vi "CustomDataHelperIAFLCytometer.vi"(0 "object in":refnum<class "AD2_DO_SDK.lvclass">, 2 "Pulse Settings":T1, 5 "error in (no error)":errorcluster) -> (14 "object out":refnum<class "AD2_DO_SDK.lvclass">, 19 "error out":errorcluster)   [LabVIEW 2019, in "AD2_DO_SDK.lvclass"]
doc: "This VI doest the same as DOconfigureCustomPattern but With a different Front panel. It is custom-made for the IAF Cytometer application"
uses:
  AD2_DO_SDK.lvclass
  DOConfigureCustomData.ctl
  DOTrigger.ctl
  AD2_WFG_SDK_class/AD2TriggerSources.ctl
  DOCustomData.ctl
  AD2_SDK_class/AD2_SDK.lvclass
panel:
  out "Numeric":i32
  out "Array 2":bool[](array[boolean])
  out "Array":bool[][](array[boolean])
  out "x*y":dbl[](array[numeric])
  # "DIO0 (camera)"
  # "DIO1 (COOL-LED CH1)"
  # "DIO2 (COOL-LED CH2)"
  # "DIO3 (COOL-LED CH1)"
  # "DIO0 Pulses at the same time as DIO1,2 and 3 +-offset"
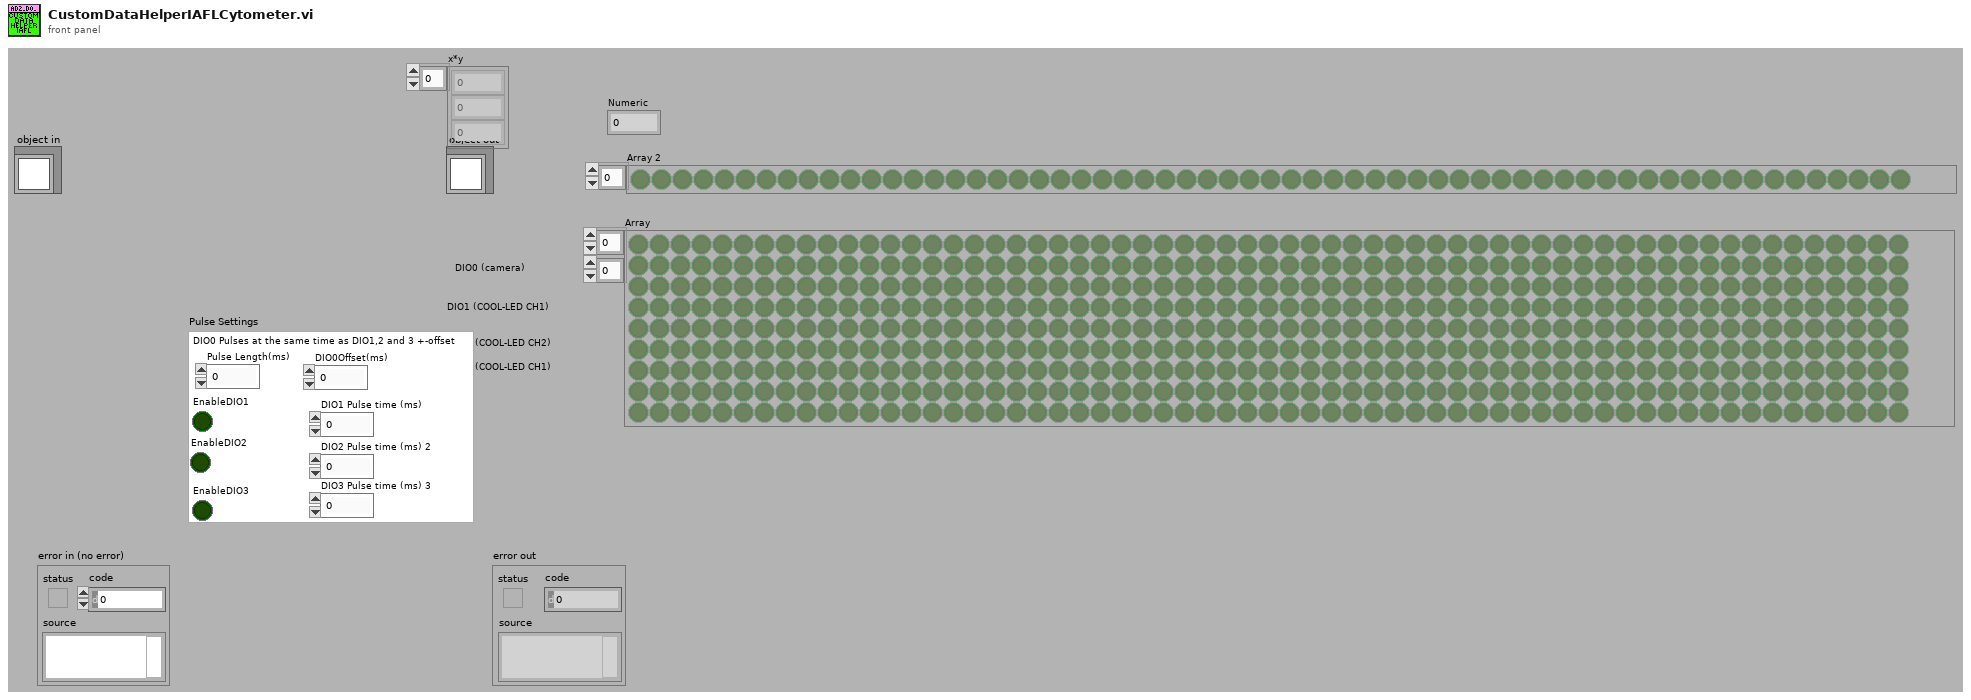
[diagram p1: front panel]
types:
  T1 = cluster{"Pulse Length(ms)":dbl, "DIO0Offset(ms)":dbl, "DIO1 Pulse time (ms)":dbl, "DIO2 Pulse time (ms) 2":dbl, "DIO3 Pulse time (ms) 3":dbl, "EnableDIO3":bool, "EnableDIO2":bool, "EnableDIO1":bool}
  T2 = typedef "AD2_SDK.lvclass/AD2TriggerSources.ctl" = enum8{"trigrsrcNone", "trigsrcPC", "trigsrcDetectorAnalogIn", "trigsrcDetectorDigitalIn", "trigsrcAnalogIn", "trigsrcDigitalIn", "trigsrcDigitalOut", "trigsrcAnalogOut1", "trigsrcAnalogOut2", "trigsrcAnalogOut3", "trigsrcAnalogOut4", "trigsrcExternal1", "trigsrcExternal2", "trigsrcExternal3", "trigsrcExternal4", ""}
  T3 = typedef "AD2_DO_SDK.lvclass/DOCustomData.ctl" = cluster{"Data":bool[], "Freq":dbl, "#Bits":u32, "Enable":bool}[]
  T4 = typedef "AD2_DO_SDK.lvclass/DOTrigger.ctl" = cluster{"secRun(0=Cont)":dbl, "secWait":dbl, "cRepeat(0=inf)":i32, "Repeat Trigger":bool, "TrigrSrc":T2}
  T5 = typedef "DOConfigureCustomData.ctl" = cluster{"DO Trigger":T4, "CustomData":T3}
  T6 = cluster{"Data":bool[], "Freq":dbl, "#Bits":u32, "Enable":bool}
  T7 = cluster{"Data":bool[], "Freq":dbl, "#Bits":u32, "Enable":bool}[]
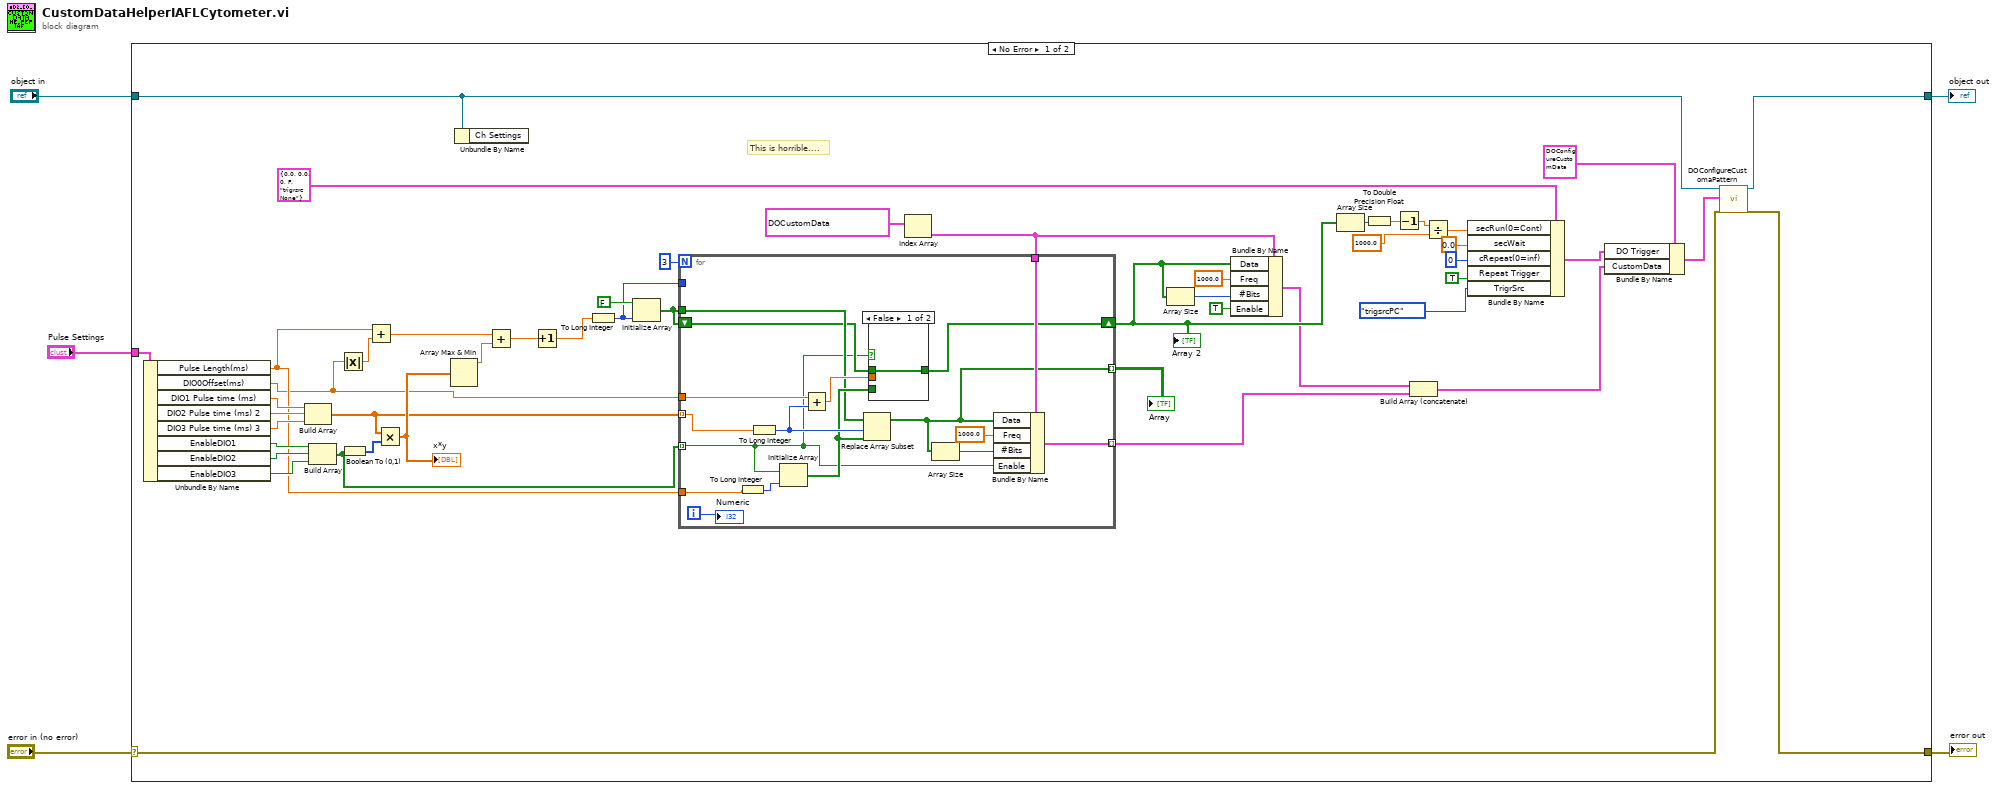
[diagram p0: block diagram]
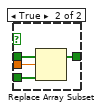
[diagram p2: hidden frame]
diagram:
  n1 = case shown="No Error" "error in (no error)" {
    selector: "error in (no error)" -> [w17 w78]
    tunnel: [w16 w78] -> w4
    tunnel: [w18 w77] -> w2
    tunnel: "object in" -> [w15 w77]
    tunnel: "Pulse Settings" -> [w49 _]
    frame No Error {
      # "This is horrible...."
      n2 = Unbundle By Name(w49) -> ("Pulse Length(ms)"=w34:dbl, "DIO0Offset(ms)"=w32:dbl, "DIO1 Pulse time (ms)"=w35:dbl, "DIO2 Pulse time (ms) 2"=w45:dbl, "DIO3 Pulse time (ms) 3"=w44:dbl, "EnableDIO1"=w48:bool, "EnableDIO2"=w47:bool, "EnableDIO3"=w46:bool)
      n3 = Build Array(w35, w45, w44) -> (w39:dbl[])
      n4 = Build Array(w48, w47, w46) -> (w38:bool[])
      n5 = Absolute Value(x=w32) -> (abs(x)=w31:dbl)
      n6 = Boolean To (0,1)(Boolean=w38) -> (0, 1=w43:i16[])
      n7 = Add(x=w34, y=w31) -> (x+y=w33:dbl)
      n8 = Multiply(x=w39, y=w43) -> (x*y=w42:dbl[])
      "x*y" <- w42
      n9 = Array Max & Min(array=w42) -> (max value=w41:dbl)  [unwired: 3 out]
      n10 = Unbundle By Name(w15) -> ()  [unwired: 1 out]
      n11 = Add(x=w33, y=w41) -> (x+y=w9:dbl)
      n12 = Increment(x=w9) -> (x+1=w8:dbl)
      n13 = To Long Integer(number=w8) -> (32bit integer=w27:i32)
      n14 = Initialize Array(FALSE, w27) -> (w36:bool[])
      n15 = Index Array(array=T3 [{"Data"=[], "Freq"=0.0, "#Bits"=0, "Enable"=FALSE}, {"Data"=[], "Freq"=0.0, "#Bits"=0, "Enable"=FALSE}, {"Data"=[], "Freq"=0.0, "#Bits"=0, "Enable"=FALSE}, {"Data"=[FALSE, FALSE, FALSE, FALSE, FALSE, FALSE, FALSE, FALSE, FALSE, FALSE, FALSE, FALSE, FALSE, FALSE, FALSE, FALSE, FALSE, FALSE, FALSE, FALSE, FALSE, FALSE, FALSE], "Freq"=0.0, "#Bits"=0, "Enable"=FALSE}, {"Data"=[], "Freq"=0.0, "#Bits"=0, "Enable"=FALSE}, {"Data"=[], "Freq"=0.0, "#Bits"=0, "Enable"=FALSE}, {"Data"=[], "Freq"=0.0, "#Bits"=0, "Enable"=FALSE}, {"Data"=[], "Freq"=0.0, "#Bits"=0, "Enable"=FALSE}, {"Data"=[], "Freq"=0.0, "#Bits"=0, "Enable"=FALSE}, {"Data"=[], "Freq"=0.0, "#Bits"=0, "Enable"=FALSE}, {"Data"=[], "Freq"=0.0, "#Bits"=0, "Enable"=FALSE}, {"Data"=[], "Freq"=0.0, "#Bits"=0, "Enable"=FALSE}, {"Data"=[], "Freq"=0.0, "#Bits"=0, "Enable"=FALSE}, {"Data"=[], "Freq"=0.0, "#Bits"=0, "Enable"=FALSE}, {"Data"=[], "Freq"=0.0, "#Bits"=0, "Enable"=FALSE}, {"Data"=[FALSE, FALSE, FALSE, FALSE, FALSE, FALSE, FALSE, FALSE, FALSE, FALSE, FALSE, FALSE, FALSE, FALSE, FALSE, FALSE, FALSE, FALSE, FALSE, FALSE, FALSE, FALSE, FALSE], "Freq"=0.0, "#Bits"=0, "Enable"=FALSE}, {"Data"=[FALSE, FALSE, FALSE, FALSE, FALSE, FALSE, FALSE, FALSE, FALSE, FALSE, FALSE, FALSE, FALSE, FALSE, FALSE, FALSE, FALSE, FALSE, FALSE, FALSE, FALSE, FALSE, FALSE], "Freq"=0.0, "#Bits"=0, "Enable"=FALSE}] ("CustomData")) -> (element=w26:T6)  [unwired: 1 in]
      n16 = for {
        N: 3 -> [_]
        tunnel: w26 -> [w63]
        tunnel: w39 -> [w56] mode=indexing
        tunnel: w38 -> [w55] mode=indexing
        tunnel: w34 -> [w71]
        tunnel: w36 -> [w65]
        shift-right: [w62] -> w23
        shift-left: w36 -> [w64]
        tunnel: w32 -> [w68]
        tunnel: w27 -> [_]
        tunnel: [w60] -> w20 mode=indexing
        tunnel: [w58] -> w6 mode=indexing
        i -> [w57]
        n17 = To Long Integer(number=w71) -> (32bit integer=w70:i32)
        n18 = To Long Integer(number=w56) -> (32bit integer=w69:i32)
        n19 = Initialize Array(w55, w70) -> (w66:bool[])
        n20 = Add(x=w68, y=w69) -> (x+y=w67:dbl)
        n21 = Replace Array Subset(array=w65, new element=w66, index=w69) -> (w58:bool[])
        n22 = case shown="False" w55 {
          tunnel: w67 -> [_ w76]
          tunnel: w66 -> [_ w75]
          tunnel: w64 -> [w72 w74]
          tunnel: [w72 w73] -> w62
          frame False {
          }
          frame True {
            n23 = Replace Array Subset(array=w74, new element=w75, index=w76) -> (w73:bool[])
          }
        }
        n24 = Array Size(array=w58) -> (size(s)=w59:i32)
        n25 = Bundle By Name(cluster=w63, "Data"=w58, "Freq"=1000.0, "#Bits"=w59, "Enable"=w55) -> (w60:T6)
        "Numeric" <- w57
      }
      "Array" <- w6
      "Array 2" <- w23
      n26 = Array Size(array=w23) -> (size(s)=w24:i32)
      n27 = Bundle By Name(cluster=w26, "Data"=w23, "Freq"=1000.0, "#Bits"=w24, "Enable"=TRUE) -> (w21:T6)
      n28 = Array Size(array=w23) -> (size(s)=w28:i32)
      n29 = To Double Precision Float(number=w28) -> (double precision float=w11:dbl)
      n30 = Decrement(x=w11) -> (x-1=w10:dbl)
      n31 = Build Array (concatenate)(w21, w20) -> (w19:T7)
      n32 = Divide(x=w10, y=1000.0) -> (x/y=w29:dbl)
      n33 = Bundle By Name(cluster=T4 {"secRun(0=Cont)"=0.0, "secWait"=0.0, "cRepeat(0=inf)"=0, "Repeat Trigger"=FALSE, "TrigrSrc"=enum."trigrsrcNone"} ("DO Trigger"), "secRun(0=Cont)"=w29, "secWait"=0.0, "cRepeat(0=inf)"=0, "Repeat Trigger"=TRUE, "TrigrSrc"=AD2TriggerSources."trigsrcPC") -> (w53:T4)
      n34 = Bundle By Name(cluster=T5 {"DO Trigger"={"secRun(0=Cont)"=0.1, "secWait"=0.0, "cRepeat(0=inf)"=0, "Repeat Trigger"=TRUE, "TrigrSrc"=enum."trigsrcPC"}, "CustomData"=[{"Data"=[FALSE, TRUE, FALSE, FALSE, FALSE, FALSE, FALSE, FALSE, FALSE, FALSE, FALSE, FALSE, TRUE, FALSE, FALSE, FALSE, FALSE, FALSE, FALSE, FALSE, FALSE, FALSE], "Freq"=1000.0, "#Bits"=1000, "Enable"=TRUE}, {"Data"=[FALSE, FALSE, FALSE, FALSE, FALSE, FALSE, FALSE, FALSE, FALSE, FALSE, FALSE, FALSE, FALSE, FALSE, FALSE, FALSE, FALSE, FALSE, FALSE, FALSE, FALSE, FALSE], "Freq"=1000.0, "#Bits"=100, "Enable"=FALSE}, {"Data"=[FALSE], "Freq"=0.0, "#Bits"=0, "Enable"=FALSE}, {"Data"=[FALSE, FALSE, FALSE, FALSE, FALSE, FALSE, FALSE, FALSE, FALSE, FALSE, FALSE, FALSE, FALSE, FALSE, FALSE, FALSE, FALSE, FALSE, FALSE, FALSE, FALSE, FALSE, FALSE], "Freq"=0.0, "#Bits"=0, "Enable"=FALSE}, {"Data"=[], "Freq"=0.0, "#Bits"=0, "Enable"=FALSE}, {"Data"=[], "Freq"=0.0, "#Bits"=0, "Enable"=FALSE}, {"Data"=[], "Freq"=0.0, "#Bits"=0, "Enable"=FALSE}, {"Data"=[], "Freq"=0.0, "#Bits"=0, "Enable"=FALSE}, {"Data"=[], "Freq"=0.0, "#Bits"=0, "Enable"=FALSE}, {"Data"=[], "Freq"=0.0, "#Bits"=0, "Enable"=FALSE}, {"Data"=[], "Freq"=0.0, "#Bits"=0, "Enable"=FALSE}, {"Data"=[], "Freq"=0.0, "#Bits"=0, "Enable"=FALSE}, {"Data"=[], "Freq"=0.0, "#Bits"=0, "Enable"=FALSE}, {"Data"=[], "Freq"=0.0, "#Bits"=0, "Enable"=FALSE}, {"Data"=[], "Freq"=0.0, "#Bits"=0, "Enable"=FALSE}, {"Data"=[FALSE, FALSE, FALSE, FALSE, FALSE, FALSE, FALSE, FALSE, FALSE, FALSE, FALSE, FALSE, FALSE, FALSE, FALSE, FALSE, FALSE, FALSE, FALSE, FALSE, FALSE, FALSE, FALSE], "Freq"=0.0, "#Bits"=0, "Enable"=FALSE}, {"Data"=[FALSE, FALSE, FALSE, FALSE, FALSE, FALSE, FALSE, FALSE, FALSE, FALSE, FALSE, FALSE, FALSE, FALSE, FALSE, FALSE, FALSE, FALSE, FALSE, FALSE, FALSE, FALSE, FALSE], "Freq"=0.0, "#Bits"=0, "Enable"=FALSE}]}, "DO Trigger"=w53, "CustomData"=w19) -> (w13:T5)
      n35 = call-dynamic "DOConfigureCustomaPattern.vi"("object in"=w15, 2:w13, "error in (no error)"=w17) -> ("object out"=w18:refnum<class "AD2_DO_SDK.lvclass">, "error out"=w16:errorcluster)  [unwired: 15 in]
    }
    frame Error {
    }
  }
  "error out" <- w4
  "object out" <- w2
